vi "Read.vi"(10 "Address":u16 format="%.0x", 11 "Memory in":refnum<class "Memory.lvclass">) -> (3 "Data Read":u8 format="%02x")   [LabVIEW 2021, in "Memory.lvclass"]
uses:
  Memory.lvclass
  Memory.lvclass/Memory.ctl
panel:
  out "Relative Index":u16 format="%.0x"
  out "Data":u8[](array[numeric]) format="%.0x"
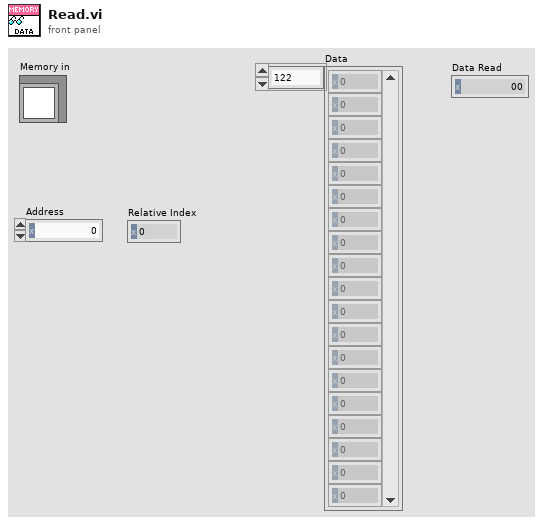
[diagram p1: front panel]
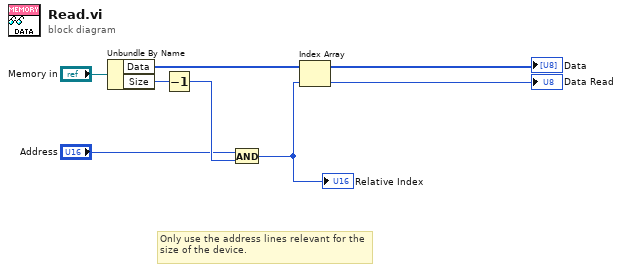
[diagram p0: block diagram]
diagram:
  # "Only use the address lines relevant for the size of the device."
  n1 = Unbundle By Name("Memory in") -> ("Data"=w6:u8[], "Size"=w4:u16)
  "Data" <- w6
  n2 = Decrement(x=w4) -> (x-1=w5:u16)
  n3 = And(x="Address", y=w5) -> (x .and. y?=w3:u16)
  "Relative Index" <- w3
  n4 = Index Array(array=w6, index=w3) -> (element=→"Data Read":u8)
